vi "SMU calibration_Auto.vi"() -> ()   [LabVIEW 2020]
uses:
  <instrlib>/Keithley 2600 Series/Public/Channel.ctl
  <vilib>/Instr/_visa.llb/VISA Configure Serial Port (Instr).vi
  <vilib>/Utility/file.llb/Read Delimited Spreadsheet (DBL).vi
  <instrlib>/Keithley 2600 Series/Keithley 2600 Series.lvlib
panel:
  out "FILE":string
  out "concatenated string":string
  out "concatenated string 4":string
  out "concatenated string 3":string
  out "concatenated string 2":string
  in  "stop":bool
  in  "Tab Control":enum32{"CONTROL", "CALIBRATION"}(tab)
  in  "String":string
  in  "set En":bool
  in  "Ring":u16(ring)=1 items=["Channel 1"=1, "Channel 2"=2, "Channel 3"=3, "Channel 4"=4]
  in  "Enable 2":bool
  out "Write \nmode":bool
  in  "Mode":bool
  in  "set mode":bool
  in  "set range":bool
  in  "Range 2":u16(ring) items=["1A", "100mA", "10mA", "1mA", "100uA", "10uA", "1uA"]
  in  "set Output":bool
  in  "Output Value":dbl format="%.3f"
  out "Unit":string
  in  "set Input":bool
  in  "Level":dbl
  out "2604B \nmode":bool
  out "Array":T1(array[cluster]) {"Output level" format="%.7f"; "Voltage" format="%.7f"; "Measurement" format="%.7f"}
  in  "VISA resource \nESP(COM4)":refnum<visa-resource-name>="COM4"
  out "calibration \nmode":bool
  in  "VISA resource \n2000(COM7)":refnum<visa-resource-name>="COM7"
  in  "VISA resource \n2604B(COM8)":refnum<visa-resource-name>="COM7"
  in  "Output File calibration":bool
  in  "Output Calibration parameter path":path
  out "Output calibration parameter":string
  out "OUTPUT_F\nmode":bool
  in  "Output FIle \nCalibation Channel":u16(ring)=1 items=["Channel 1"=1, "Channel 2"=2, "Channel 3"=3, "Channel 4"=4]
  in  "Input File calibration":bool
  in  "Input Calibration parameter path  - Voltage":path
  out "Input calibration parameter":string
  out "INPUT_F\nmode":bool
  in  "Input FIle \nCalibation Channel":u16(ring)=1 items=["Channel 1"=1, "Channel 2"=2, "Channel 3"=3, "Channel 4"=4]
  in  "Input Calibration parameter path  - Current":path
  out "CH1 Calibration TX":string
  out "CH2 Calibration TX":string
  out "CH3 Calibration TX":string
  out "CH4 Calibration TX":string
  out "CH1\nCali mode":bool
  out "CH4\nCali mode":bool
  in  "calibration 4":bool
  out "CH3\nCali mode":bool
  in  "calibration 3":bool
  out "CH2\nCali mode":bool
  in  "calibration 2":bool
  in  "calibration 1":bool
  in  "Channel (Channel A)":T2
  out "STOP LED":bool
  out "tmp data":string
  out "Array 3":bool[](array[boolean])
  out "Array 2":i32[](array[numeric])
  out "test":bool
  out "extra buffer":string
  out "Range":string
  out "VI mode":string
  out "Enable":string
  out "Current":dbl
  out "Voltage":dbl
  out "Output level":dbl
  out "SMU Channel":string
  # "made by Ji Won Kim  2021.03.16"
  # "SOURCE MEASUREMENT SYSTEM"
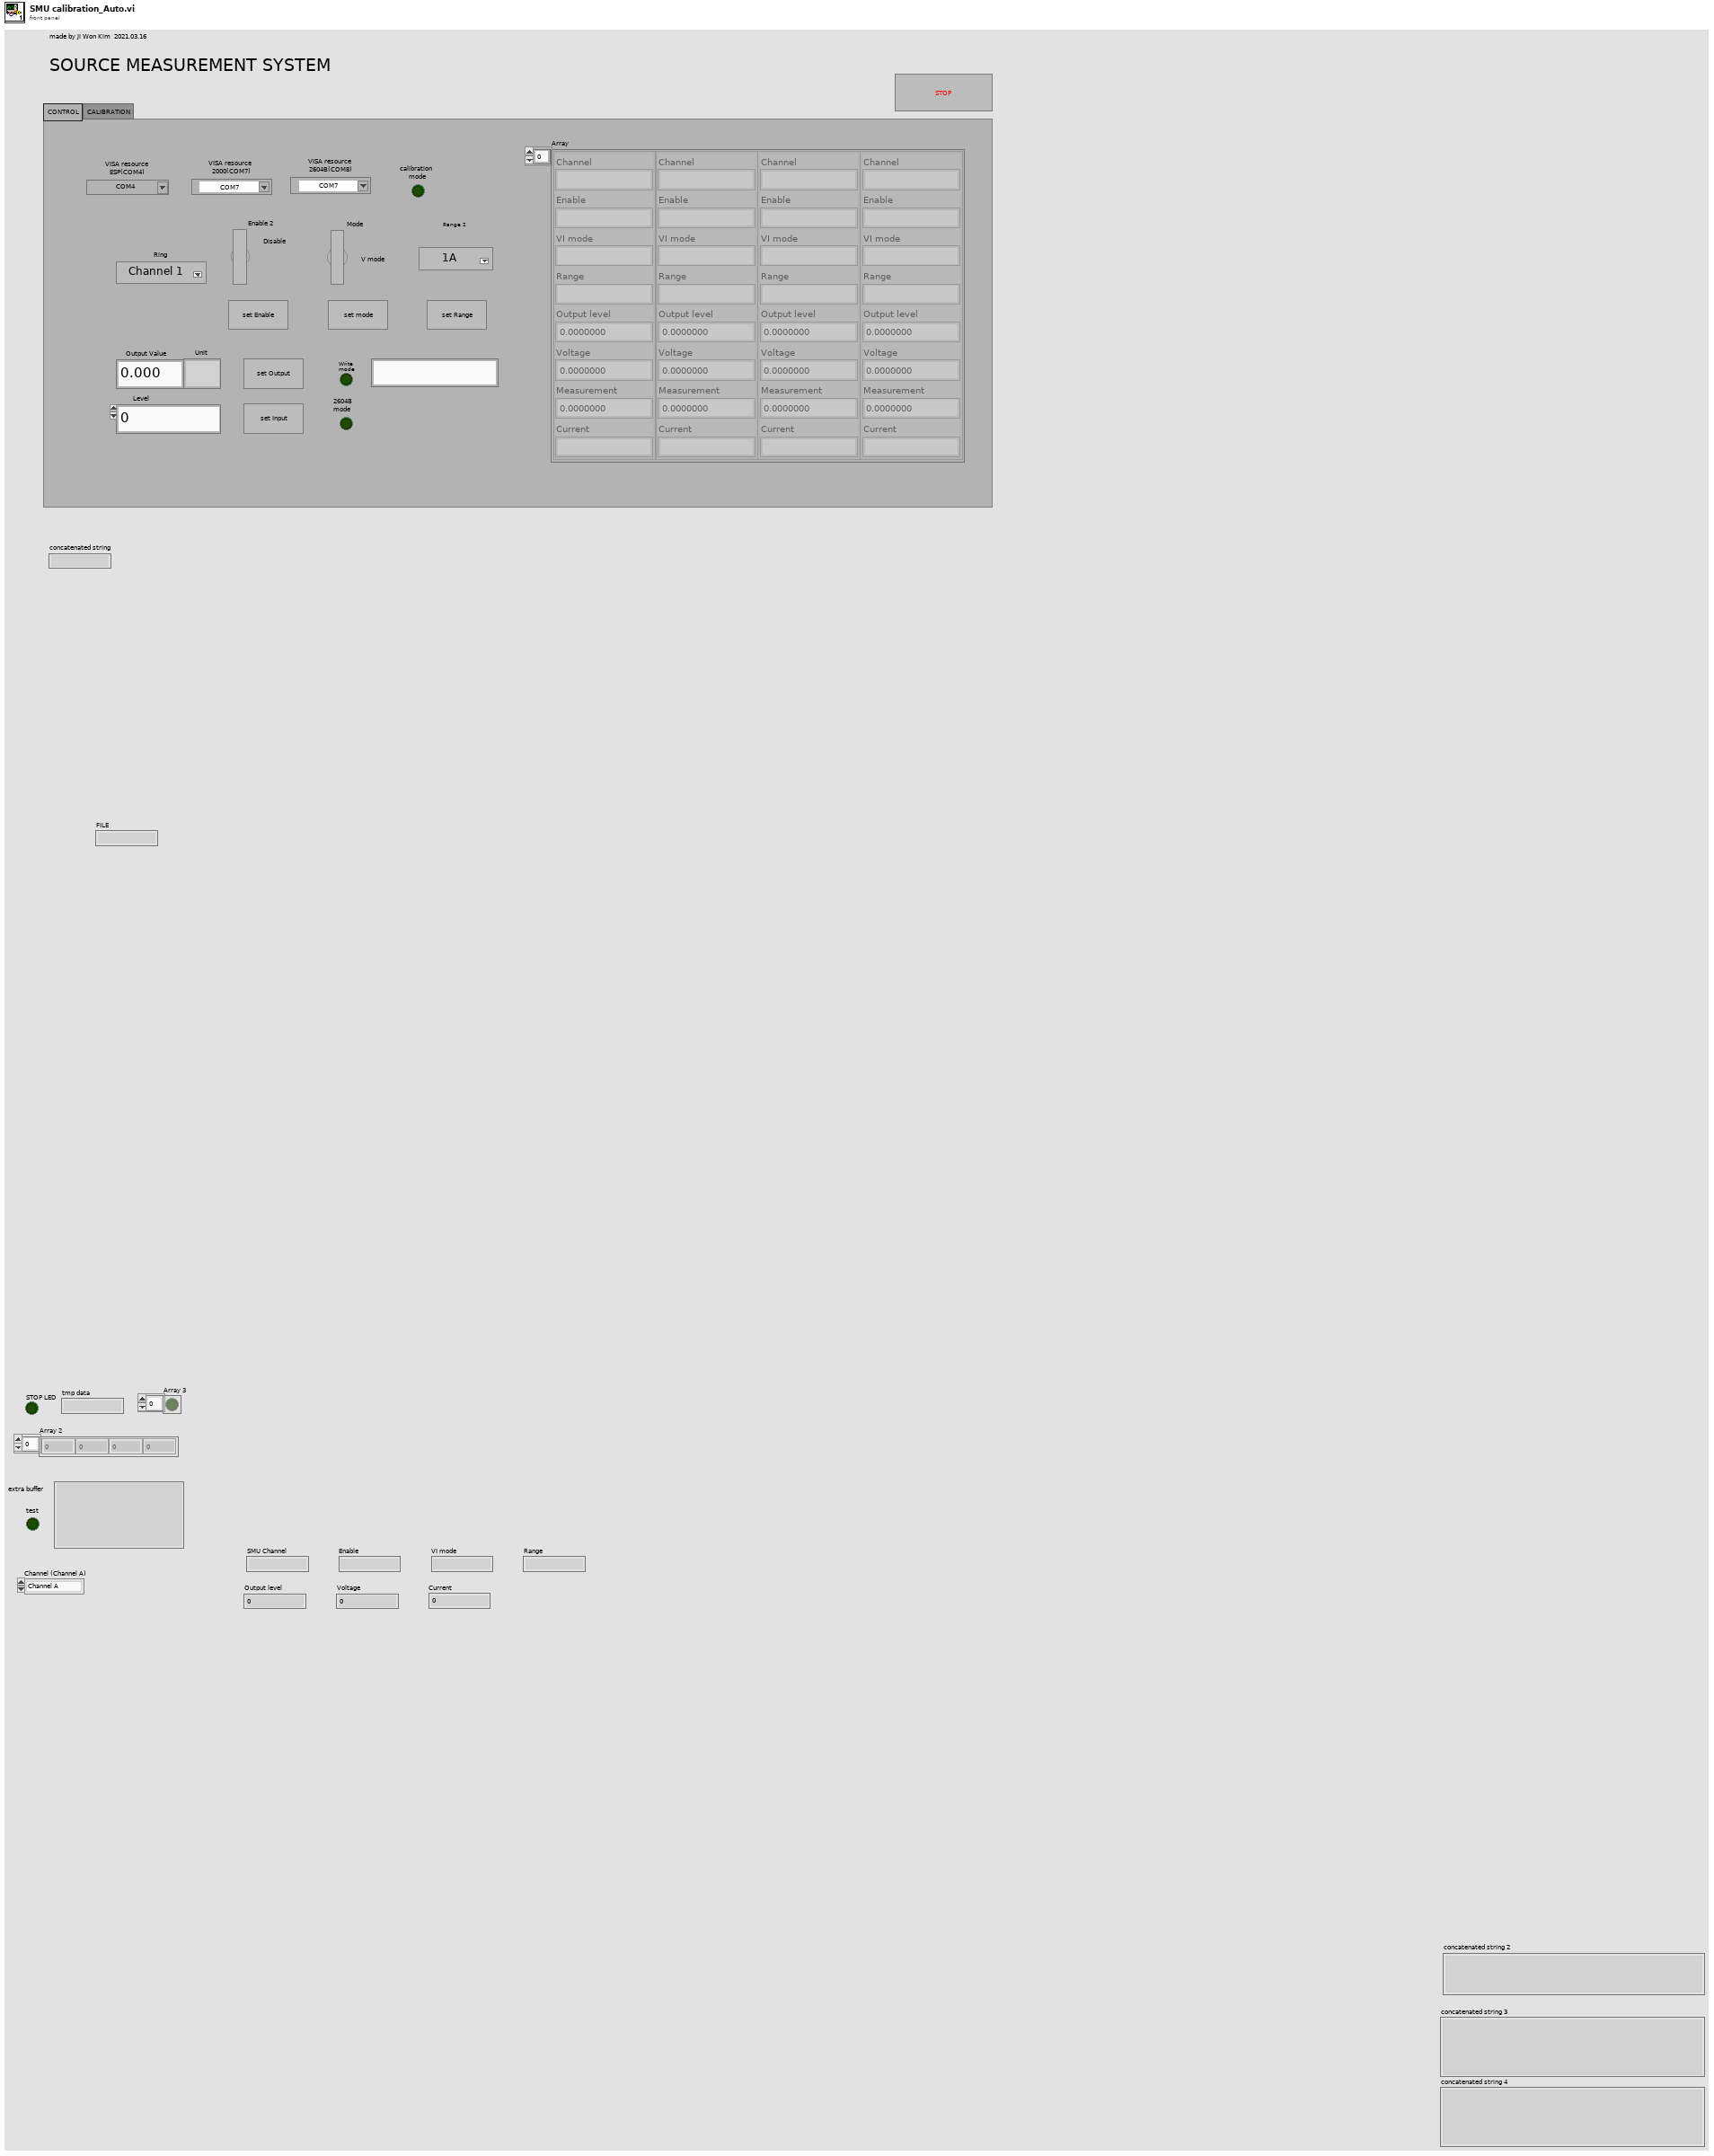
[diagram p1: front panel]
types:
  T1 = cluster{"Channel":string, "Enable":string, "VI mode":string, "Range":string, "Output level":dbl, "Voltage":dbl, "Measurement":dbl, "Current":string}[]
  T2 = typedef "Keithley 2600 Series.lvlib/Channel.ctl" = enum32{"Channel A", "Channel B"}
  T3 = cluster{"Baud Rate":u32, "Parity":u16, "Data Bits":u16, "Stop Bits":u16, "Flow Control":u16}
  T4 = cluster{"trimmed string":string, "Enable":string, "VI mode":string, "output string":string, dbl, dbl, dbl, string}
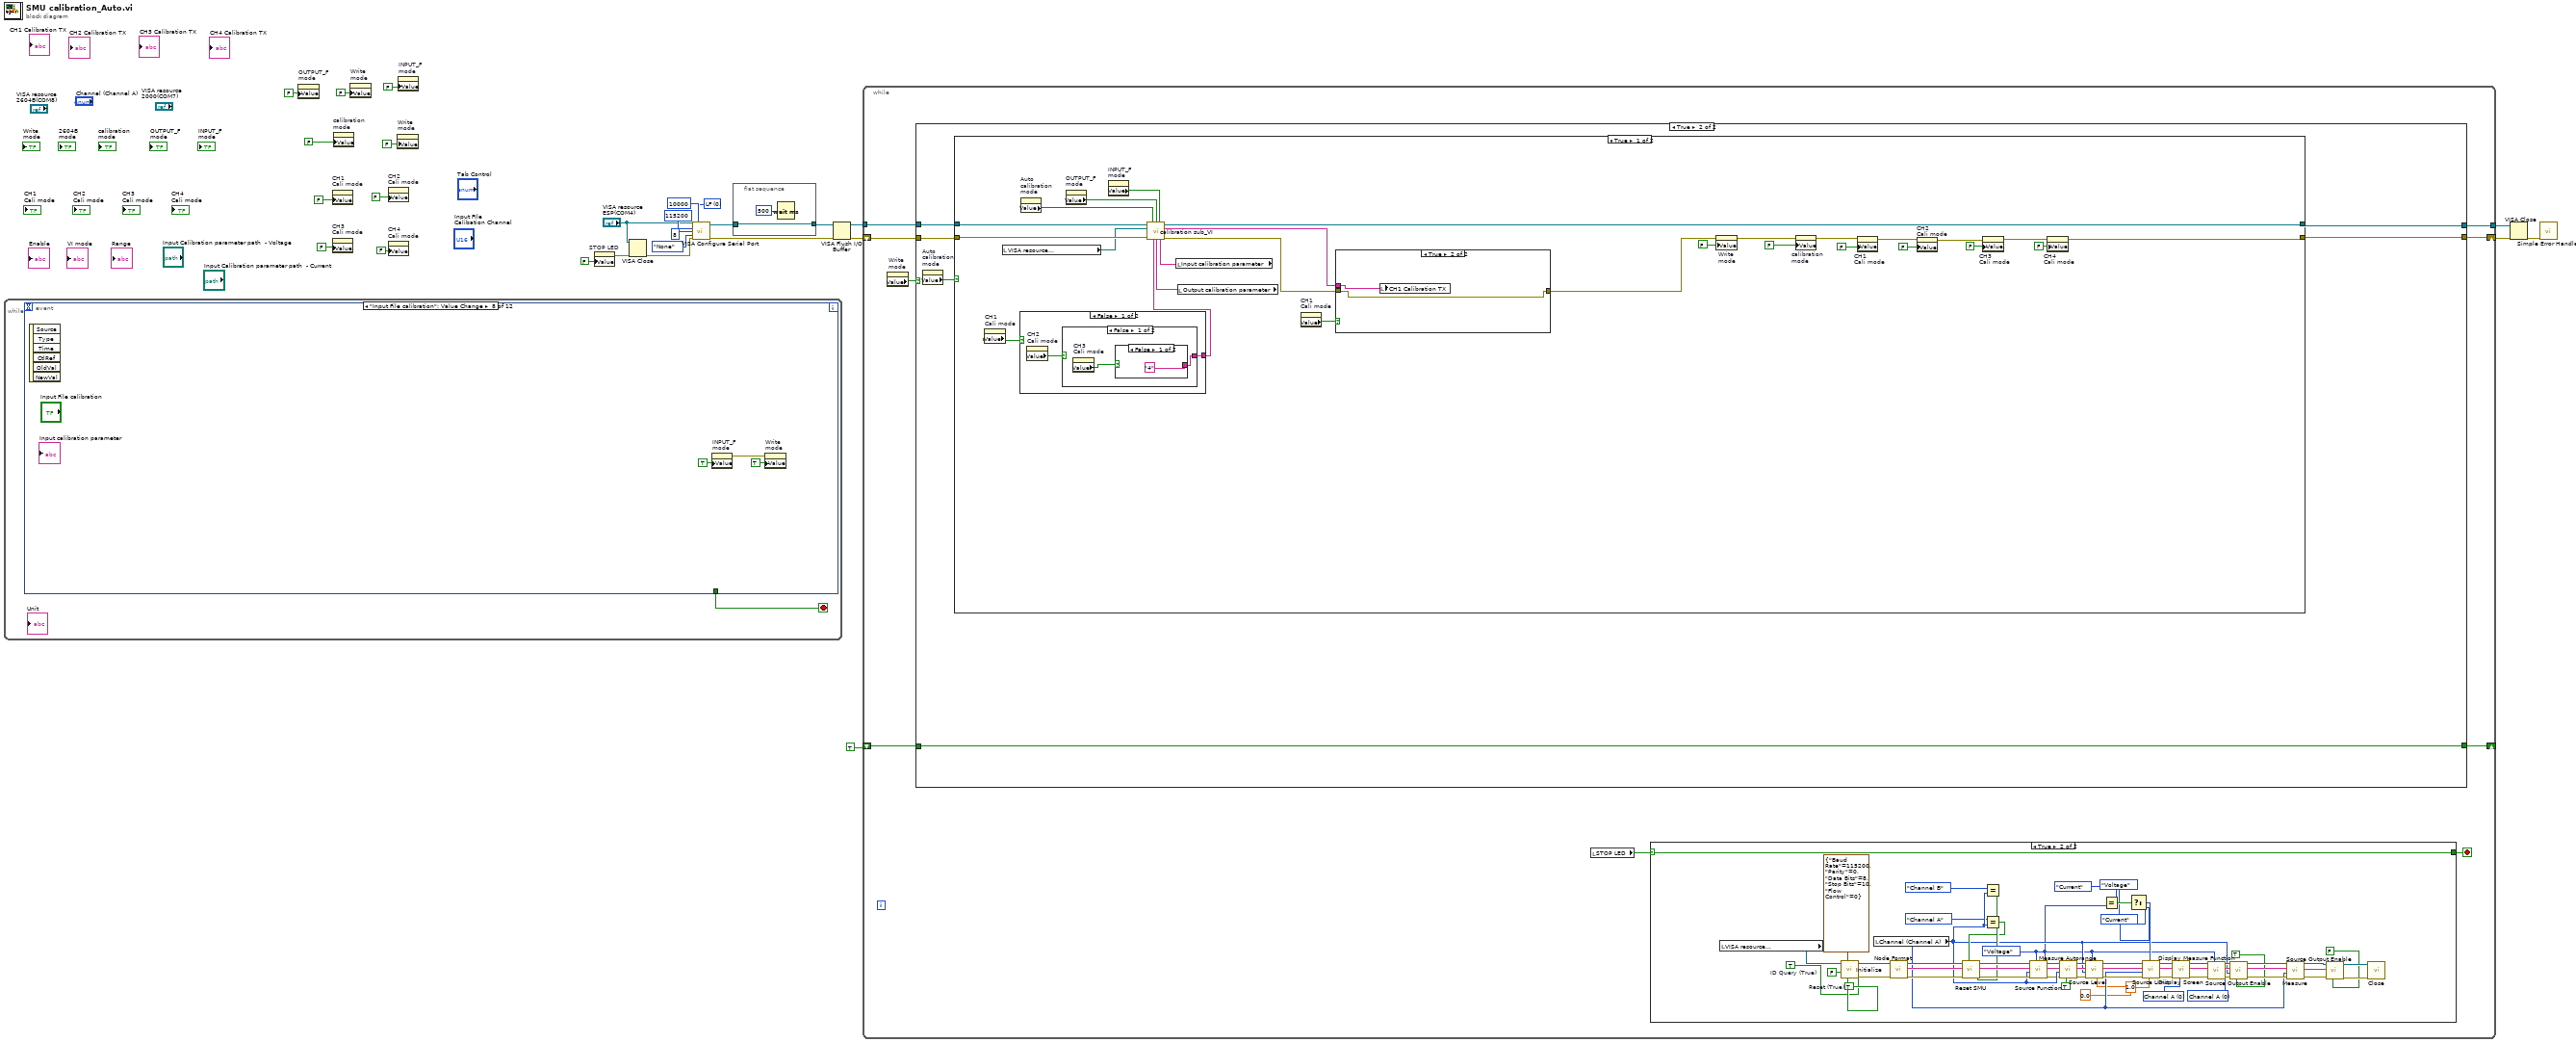
[diagram p0: block diagram]
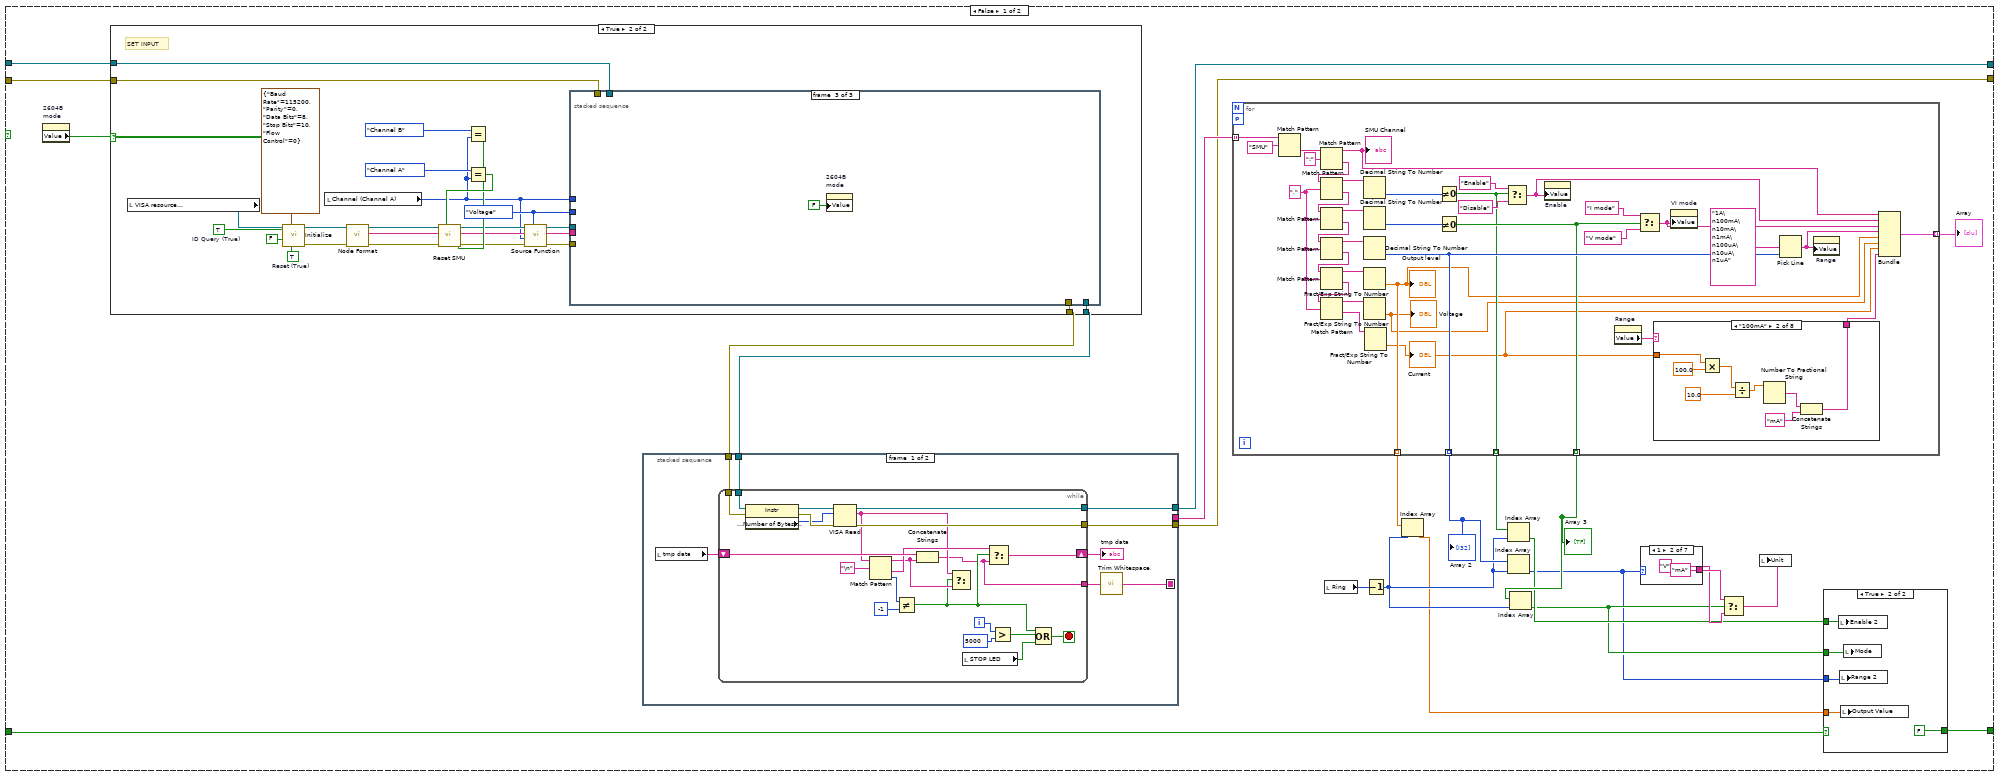
[diagram p2: hidden frame]
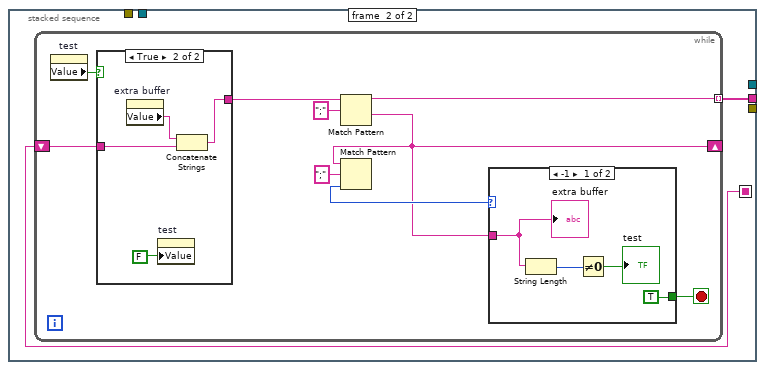
[diagram p3: hidden frame]
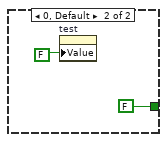
[diagram p5: hidden frame]
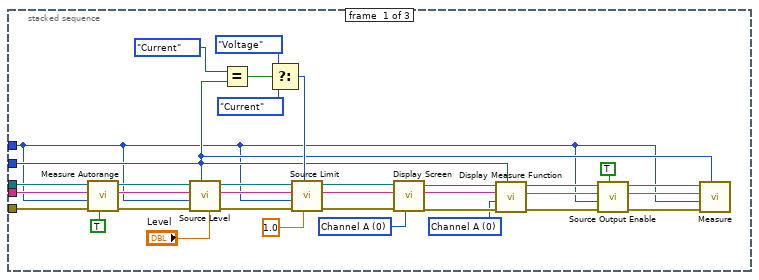
[diagram p7: hidden frame]
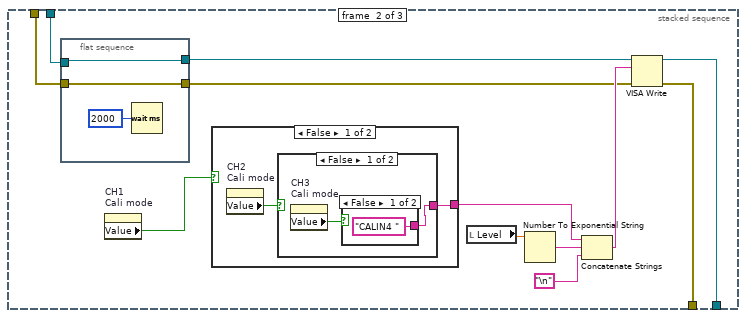
[diagram p8: hidden frame]
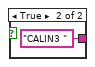
[diagram p9: hidden frame]
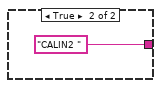
[diagram p10: hidden frame]
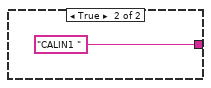
[diagram p11: hidden frame]
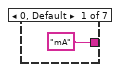
[diagram p13: hidden frame]
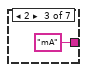
[diagram p14: hidden frame]
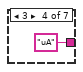
[diagram p15: hidden frame]
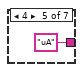
[diagram p16: hidden frame]
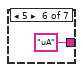
[diagram p17: hidden frame]
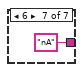
[diagram p18: hidden frame]
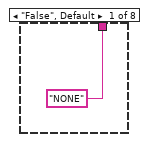
[diagram p19: hidden frame]
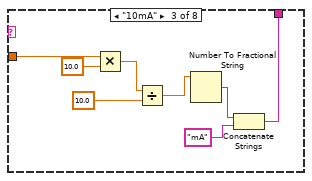
[diagram p20: hidden frame]
diagram:
  w25 = u16 0 items=["LF"]
  n1 = while {
    stop <- w28 stop-if-true
    n2 = event shown="[7] \"Input File calibration\": Value Change" {
      selector: _ -> [_ _ _ _ _ _ _ _ _ _ _ _]
      dyn-events: _ -> [_ _ _ _ _ _ _ _ _ _ _ _]
      timeout: _ -> [_ _ _ _ _ _ _ _ _ _ _ _]
      tunnel: [w29 _ _ _ _ _ _ _ _ _ _ _] -> w28
      event "stop": Value Change {
        n3 = event-data() -> ("NewVal"=w29:bool)  [unwired: 1 in, 5 out]
        "STOP LED" <- w29
      }
      event "set En": Value Change {
        n4 = event-data() -> ()  [unwired: 1 in, 6 out]
        n5 = Boolean To (0,1)(Boolean="Enable 2") -> (0, 1=w41:i16)
        n6 = Number To Decimal String(number="Ring", width (-)=i16 1) -> (decimal integer string=w39:string)
        n7 = Number To Decimal String(number=w41, width (-)=i16 1) -> (decimal integer string=w42:string)
        n8 = Concatenate Strings("ENA", w39, " " ("string"), w42, "\n") -> (w30:string)
        n9 = property on="String" class="Str"("Value"=w30) -> (error out=w32:errorcluster)  [unwired: 2 in, 1 out]
        n10 = property on="Write \nmode" class="Bool (strict)"(error in=w32, "Value"=TRUE ("Write mode")) -> ()  [unwired: 1 in, 2 out]
      }
      event "set mode": Value Change {
        n11 = event-data() -> ()  [unwired: 1 in, 6 out]
        n12 = local read "Ring"() -> (w55:u16)
        n13 = Boolean To (0,1)(Boolean="Mode") -> (0, 1=w53:i16)
        n14 = Number To Decimal String(number=w55, width (-)=i16 1) -> (decimal integer string=w51:string)
        n15 = Number To Decimal String(number=w53, width (-)=i16 1) -> (decimal integer string=w54:string)
        n16 = Concatenate Strings("VIM", w51, " " ("string"), w54, "\n") -> (w49:string)
        n17 = property on="String" class="Str"("Value"=w49) -> (error out=w50:errorcluster)  [unwired: 2 in, 1 out]
        n18 = property on="Write \nmode" class="Bool (strict)"(error in=w50, "Value"=TRUE ("Write mode")) -> ()  [unwired: 1 in, 2 out]
      }
      event "set range": Value Change {
        n19 = event-data() -> ()  [unwired: 1 in, 6 out]
        n20 = local read "Ring"() -> (w66:u16)
        n21 = Number To Decimal String(number=w66, width (-)=i16 1) -> (decimal integer string=w64:string)
        n22 = Number To Decimal String(number="Range 2", width (-)=i16 1) -> (decimal integer string=w65:string)
        n23 = Concatenate Strings("RAN", w64, " " ("string"), w65, "\n") -> (w62:string)
        n24 = property on="String" class="Str"("Value"=w62) -> (error out=w63:errorcluster)  [unwired: 2 in, 1 out]
        n25 = property on="Write \nmode" class="Bool (strict)"(error in=w63, "Value"=TRUE ("Write mode")) -> ()  [unwired: 1 in, 2 out]
      }
      event "set Output": Value Change {
        n26 = event-data() -> ()  [unwired: 1 in, 6 out]
        n27 = local read "Ring"() -> (w76:u16)
        n28 = local read "Array 2"() -> (w75:i32[])
        n29 = Decrement(x=w76) -> (x-1=w69:u16)
        n30 = Index Array(array=w75, index=w69) -> (element=w74:i32)
        n31 = case shown="0, Default" w74 {
          tunnel: [1000.0 100.0 10.0 1000.0 100.0 10.0 1.0] -> w77
          frame 0, Default {
          }
          frame 1 {
          }
          frame 2 {
          }
          frame 3 {
          }
          frame 4 {
          }
          frame 5 {
          }
          frame 6 {
          }
        }
        n32 = local read "Array 3"() -> (w71:bool[])
        n33 = Index Array(array=w71, index=w69) -> (element=w70:bool)
        n34 = Divide(x="Output Value", y=w77) -> (x/y=w78:dbl)
        n35 = Multiply(x=w78, y=10.0) -> (x*y=w73:dbl)
        n36 = Select(t=w73, s=w70, f="Output Value") -> (s? t:f=w68:dbl)
        n37 = local read "Ring"() -> (w89:u16)
        n38 = Number To Fractional String(number=w68, precision (6)=i16 4) -> (F-format string=w90:string)  [unwired: 2 in]
        n39 = Number To Decimal String(number=w89, width (-)=i16 1) -> (decimal integer string=w88:string)
        n40 = Concatenate Strings("CAL", w88, " " ("string"), w90, "\n") -> (w86:string)
        n41 = property on="String" class="Str"("Value"=w86) -> (error out=w87:errorcluster)  [unwired: 2 in, 1 out]
        n42 = property on="Write \nmode" class="Bool (strict)"(error in=w87, "Value"=TRUE ("Write mode")) -> ()  [unwired: 1 in, 2 out]
      }
      event "set Input": Value Change {
        n43 = event-data() -> ()  [unwired: 1 in, 6 out]
        n44 = property on="2604B \nmode" class="Bool (strict)"("Value"=TRUE ("2604B mode")) -> ()  [unwired: 2 in, 2 out]
      }
      event "Output File calibration": Value Change {
        n45 = event-data() -> ()  [unwired: 1 in, 6 out]
        n46 = call-poly <vilib>:"Read Delimited Spreadsheet.vi"("file path (dialog if empty)"="Output Calibration parameter path", "delimiter (\\t)"="," ("delimiter (\\t)")) -> ("all rows"=w111:dbl[][])  [unwired: 8 in, 5 out]
        n47 = Index Array(array=w111, index (col)=1 ("disabled index (col)")) -> (element=w115:dbl[])  [unwired: 1 in]
        n48 = Array To Spreadsheet String(delimiter (Tab)=",", array=w115, 3:"%5.3f" ("format string")) -> (spreadsheet string=w109:string)
        n49 = Number To Decimal String(number="Output FIle \nCalibation Channel", width (-)=i16 1) -> (decimal integer string=w100:string)
        n50 = call <vilib>:"Trim Whitespace.vi"("string"=w109) -> ("trimmed string"=w108:string)  [unwired: 1 in]
        n51 = Concatenate Strings("DAQ" ("string"), w100, " " ("string"), "-10,-9,-8,-7,-6,-5,-4,-3,-2,-1,0,1,2,3,4,5,6,7,8,9,10" ("string"), ";" ("string"), w108, "\n") -> (w107:string)
        n52 = Concatenate Strings(w107, "\n") -> (w118:string)
        n53 = property on="Output calibration parameter" class="Str"("Value"=w118) -> (error out=w121:errorcluster)  [unwired: 2 in, 1 out]
        n54 = property on="OUTPUT_F\nmode" class="Bool (strict)"(error in=w121, "Value"=TRUE ("calibration mode 2")) -> (error out=w119:errorcluster)  [unwired: 1 in, 1 out]
        n55 = property on="Write \nmode" class="Bool (strict)"(error in=w119, "Value"=TRUE ("Write mode")) -> ()  [unwired: 1 in, 2 out]
      }
      event "Input File calibration": Value Change {
        n56 = event-data() -> ()  [unwired: 1 in, 6 out]
        n57 = property on="INPUT_F\nmode" class="Bool (strict)"("Value"=TRUE ("calibration mode 2")) -> (error out=w123:errorcluster)  [unwired: 2 in, 1 out]
        n58 = property on="Write \nmode" class="Bool (strict)"(error in=w123, "Value"=TRUE ("Write mode")) -> ()  [unwired: 1 in, 2 out]
      }
      event "calibration 1": Value Change {
        n59 = event-data() -> ()  [unwired: 1 in, 6 out]
        n60 = property on="calibration \nmode" class="Bool (strict)"("Value"=TRUE ("Write mode")) -> (error out=w128:errorcluster)  [unwired: 2 in, 1 out]
        n61 = property on="Write \nmode" class="Bool (strict)"(error in=w128, "Value"=TRUE ("Write mode")) -> (error out=w127:errorcluster)  [unwired: 1 in, 1 out]
        n62 = property on="CH1\nCali mode" class="Bool (strict)"(error in=w127, "Value"=TRUE ("Write mode")) -> ()  [unwired: 1 in, 2 out]
      }
      event "calibration 2": Value Change {
        n63 = event-data() -> ()  [unwired: 1 in, 6 out]
        n64 = property on="calibration \nmode" class="Bool (strict)"("Value"=TRUE ("Write mode")) -> (error out=w133:errorcluster)  [unwired: 2 in, 1 out]
        n65 = property on="Write \nmode" class="Bool (strict)"(error in=w133, "Value"=TRUE ("Write mode")) -> (error out=w132:errorcluster)  [unwired: 1 in, 1 out]
        n66 = property on="CH2\nCali mode" class="Bool (strict)"(error in=w132, "Value"=TRUE ("Write mode")) -> ()  [unwired: 1 in, 2 out]
      }
      event "calibration 3": Value Change {
        n67 = event-data() -> ()  [unwired: 1 in, 6 out]
        n68 = property on="calibration \nmode" class="Bool (strict)"("Value"=TRUE ("Write mode")) -> (error out=w138:errorcluster)  [unwired: 2 in, 1 out]
        n69 = property on="Write \nmode" class="Bool (strict)"(error in=w138, "Value"=TRUE ("Write mode")) -> (error out=w137:errorcluster)  [unwired: 1 in, 1 out]
        n70 = property on="CH3\nCali mode" class="Bool (strict)"(error in=w137, "Value"=TRUE ("Write mode")) -> ()  [unwired: 1 in, 2 out]
      }
      event "calibration 4": Value Change {
        n71 = event-data() -> ()  [unwired: 1 in, 6 out]
        n72 = property on="calibration \nmode" class="Bool (strict)"("Value"=TRUE ("Write mode")) -> (error out=w143:errorcluster)  [unwired: 2 in, 1 out]
        n73 = property on="Write \nmode" class="Bool (strict)"(error in=w143, "Value"=TRUE ("Write mode")) -> (error out=w142:errorcluster)  [unwired: 1 in, 1 out]
        n74 = property on="CH4\nCali mode" class="Bool (strict)"(error in=w142, "Value"=TRUE ("Write mode")) -> ()  [unwired: 1 in, 2 out]
      }
    }
  }
  n75 = property on="OUTPUT_F\nmode" class="Bool (strict)"("Value"=FALSE ("calibration mode 2")) -> ()  [unwired: 2 in, 2 out]
  n76 = property on="CH1\nCali mode" class="Bool (strict)"("Value"=FALSE ("Write mode")) -> ()  [unwired: 2 in, 2 out]
  n77 = property on="CH3\nCali mode" class="Bool (strict)"("Value"=FALSE ("calibration \nmode 3")) -> ()  [unwired: 2 in, 2 out]
  n78 = property on="calibration \nmode" class="Bool (strict)"("Value"=FALSE ("calibration mode")) -> ()  [unwired: 2 in, 2 out]
  n79 = property on="Write \nmode" class="Bool (strict)"("Value"=FALSE ("Write mode")) -> ()  [unwired: 2 in, 2 out]
  n80 = property on="CH2\nCali mode" class="Bool (strict)"("Value"=FALSE ("calibration \nmode 2")) -> ()  [unwired: 2 in, 2 out]
  n81 = property on="CH4\nCali mode" class="Bool (strict)"("Value"=FALSE ("calibration \nmode 4")) -> ()  [unwired: 2 in, 2 out]
  n82 = property on="Write \nmode" class="Bool (strict)"("Value"=FALSE ("Write mode")) -> ()  [unwired: 2 in, 2 out]
  n83 = property on="INPUT_F\nmode" class="Bool (strict)"("Value"=FALSE ("Write mode")) -> ()  [unwired: 2 in, 2 out]
  n84 = property on="STOP LED" class="Bool (strict)"("Value"=FALSE ("NewVal")) -> (error out=w11:errorcluster)  [unwired: 2 in, 1 out]
  n85 = VISA Close(VISA resource name="VISA resource \nESP(COM4)", error in (no error)=w11) -> (error out=w13:errorcluster)
  n86 = call-poly "VISA Configure Serial Port"("VISA resource name"="VISA resource \nESP(COM4)", "timeout (10sec)"=u32 10000, "termination char\n(0xA = '\\n' = LF)"=w25, "baud rate (9600)"=u32 115200, "data bits (8)"=u16 8, "parity (0:none)"=enum16{"None", "Odd", "Even", "Mark", "Space"}."None", "error in (no error)"=w13) -> ("VISA resource name out"=w19:refnum<visa-resource-name>, "error out"=w17:errorcluster)  [unwired: 7 in]
  n87 = flat-sequence {
    tunnel: [w146] -> w18
    tunnel: w19 -> [w146]
    frame #0 {
      n88 = Wait (ms)(milliseconds to wait=u32 500 ("대기 시간(ms)")) -> ()  [unwired: 1 out]
    }
  }
  n89 = VISA Flush I/O Buffer(VISA resource name=w18, error in (no error)=w17) -> (VISA resource name out=w15:refnum<visa-resource-name>, error out=w16:errorcluster)  [unwired: 1 in]
  n90 = while {
    tunnel: [w156] -> w27
    shift-right: [w152] -> w21
    shift-left: w16 -> [w151]
    tunnel: w15 -> [w155]
    shift-right: [w153] -> _
    shift-left: TRUE -> [w154]
    stop <- w149 stop-if-true
    n91 = property on="Write \nmode" class="Bool (strict)"() -> ("Value"=w148:bool)  [unwired: 2 in, 2 out]
    n92 = case shown="True" w148 {
      tunnel: [w157 w427] -> w152
      tunnel: [w158 w428] -> w156
      tunnel: w155 -> [w164 w429]
      tunnel: w154 -> [w167 w426]
      tunnel: [w166 w426] -> w153
      tunnel: w151 -> [w163 w424]
      frame False {
        n93 = property on="2604B \nmode" class="Bool (strict)"() -> ("Value"=w162:bool)  [unwired: 2 in, 2 out]
        n94 = case shown="True" w162 {
          tunnel: w164 -> [w234 w259]
          tunnel: w163 -> [w233 w258]
          tunnel: [w234 w235] -> w160
          tunnel: [w233 w236] -> w161
          frame False {
          }
          frame True {
            w240 = enum32{"Current", "Voltage"}."Voltage" ("Source Function (Current)")
            w256 = TRUE  # Reset (True)
            w257 = TRUE  # ID Query (True)
            # "SET INPUT"
            n95 = local read "VISA resource \n2604B(COM8)"() -> (w238:refnum<visa-resource-name>)
            n96 = call <instrlib>:"Initialize.vi"("Reset (True)"=w256, "Serial Configuration"=T3 {"Baud Rate"=115200, "Parity"=0, "Data Bits"=8, "Stop Bits"=10, "Flow Control"=0}, "Error Query (False)"=FALSE, "ID Query (True)"=w257, "VISA resource name"=w238) -> ("error out"=w245:errorcluster, "VISA resource name out"=w254:refnum<visa-resource-name>)  [unwired: 1 in, 4 out]
            n97 = local read "Channel (Channel A)"() -> (w237:T2)
            n98 = call <instrlib>:"Node Format.vi"("error in"=w245) -> ("error out"=w244:errorcluster, "Formatted Node"=w246:string)  [unwired: 1 in, 8 out]
            n99 = Equal?(x=enum32{"Channel A", "Channel B"}."Channel B", y=w237) -> (x = y?=w250:bool)
            n100 = Equal?(x=enum32{"Channel A", "Channel B"}."Channel A", y=w237) -> (x = y?=w251:bool)
            n101 = call <instrlib>:"Reset SMU.vi"("SMU B (No)"=w250, "SMU A (No)"=w251, "error in (no error)"=w244, "Node In"=w246, "VISA resource name"=w254) -> ("error out"=w249:errorcluster, "Node Out"=w247:string, "VISA resource name out"=w248:refnum<visa-resource-name>)  [unwired: 4 out]
            n102 = call <instrlib>:"Source Function.vi"("Function (Current)"=w240, "error in (no error)"=w249, "Channel (Channel A)"=w237, "Node In"=w247, "VISA resource name"=w248) -> ("error out"=w241:errorcluster, "Node Out"=w243:string, "VISA resource name out"=w242:refnum<visa-resource-name>)  [unwired: 4 out]
            n103 = stacked-sequence {
              tunnel: w243 -> [w264 _ _]
              tunnel: w242 -> [w267 _ _]
              tunnel: w241 -> [w263 _ _]
              tunnel: w237 -> [w261 _ _]
              tunnel: w240 -> [w270 _ _]
              tunnel: w259 -> [_ w305 _]
              tunnel: w258 -> [_ w304 _]
              tunnel: [_ w297 _] -> w235
              tunnel: [_ w296 _] -> w236
              frame #0 {
                w271 = u16 0 items=["Channel A", "Channel B"] ("Channel (Channel A)")
                w281 = u16 0 items=["Channel A", "Channel B", "Channels A & B", "User"] ("Screen (Channels A & B)")
                n104 = call <instrlib>:"Measure Autorange.vi"("Autorange (On)"=TRUE, "error in (no error)"=w263, "Channel (Channel A)"=w261, "Node In"=w264, "VISA resource name"=w267) -> ("error out"=w262:errorcluster, "Node Out"=w265:string, "VISA resource name out"=w266:refnum<visa-resource-name>)  [unwired: 3 in, 1 out]
                n105 = call <instrlib>:"Source Level.vi"("Level (0.000)"="Level", "Function (Current)"=w270, "error in (no error)"=w262, "Channel (Channel A)"=w261, "Node In"=w265, "VISA resource name"=w266) -> ("error out"=w293:errorcluster, "Node Out"=w288:string, "VISA resource name out"=w292:refnum<visa-resource-name>)  [unwired: 3 out]
                n106 = Equal?(x=enum32{"Current", "Voltage"}."Current", y=w270) -> (x = y?=w285:bool)
                n107 = Select(t=enum32{"Current", "Voltage"}."Voltage" ("x"), s=w285, f=enum32{"Current", "Voltage"}."Current") -> (s? t:f=w283:enum32{"Current", "Voltage"})
                n108 = call <instrlib>:"Source Limit.vi"("Limit (0.000)"=1.0, "Function (Current)"=w283, "error in (no error)"=w293, "Channel (Channel A)"=w261, "Node In"=w288, "VISA resource name"=w292) -> ("error out"=w278:errorcluster, "Node Out"=w279:string, "VISA resource name out"=w280:refnum<visa-resource-name>)  [unwired: 3 out]
                n109 = call <instrlib>:"Display Screen.vi"("Screen (Channels A & B)"=w281, "error in (no error)"=w278, "Node In"=w279, "VISA resource name"=w280) -> ("error out"=w275:errorcluster, "Node Out"=w276:string, "VISA resource name out"=w277:refnum<visa-resource-name>)  [unwired: 4 in, 1 out]
                n110 = call <instrlib>:"Display Measure Function.vi"("Function (Current)"=w270, "error in (no error)"=w275, "Channel (Channel A)"=w271, "Node In"=w276, "VISA resource name"=w277) -> ("error out"=w272:errorcluster, "Node Out"=w273:string, "VISA resource name out"=w274:refnum<visa-resource-name>)  [unwired: 3 in, 1 out]
                n111 = call <instrlib>:"Source Output Enable.vi"("Output (Off)"=TRUE, "error in (no error)"=w272, "Channel (Channel A)"=w261, "Node In"=w273, "VISA resource name"=w274) -> ("error out"=w291:errorcluster, "Node Out"=w287:string, "VISA resource name out"=w290:refnum<visa-resource-name>)  [unwired: 4 out]
                n112 = call <instrlib>:"Measure.vi"("Function (Current)"=w270, "error in (no error)"=w291, "Channel (Channel A)"=w261, "Node In"=w287, "VISA resource name"=w290) -> ()  [unwired: 2 in, 5 out]
              }
              frame #1 {
                n113 = flat-sequence {
                  tunnel: w305 -> [w316]
                  tunnel: [w316] -> w299
                  tunnel: w304 -> [w315]
                  tunnel: [w315] -> w298
                  frame #0 {
                    n114 = Wait (ms)(milliseconds to wait=u32 2000) -> ()  [unwired: 1 out]
                  }
                }
                n115 = property on="CH1\nCali mode" class="Bool (strict)"() -> ("Value"=w295:bool)  [unwired: 2 in, 2 out]
                n116 = case shown="False" w295 {
                  tunnel: [w306 "CALIN1 " ("string")] -> w294
                  frame False {
                    n117 = property on="CH2\nCali mode" class="Bool (strict)"() -> ("Value"=w307:bool)  [unwired: 2 in, 2 out]
                    n118 = case shown="False" w307 {
                      tunnel: [w308 "CALIN2 " ("string")] -> w306
                      frame False {
                        n119 = property on="CH3\nCali mode" class="Bool (strict)"() -> ("Value"=w309:bool)  [unwired: 2 in, 2 out]
                        n120 = case shown="False" w309 {
                          tunnel: ["CALIN4 " ("string") "CALIN3 " ("string")] -> w308
                          frame False {
                          }
                          frame True {
                          }
                        }
                      }
                      frame True {
                      }
                    }
                  }
                  frame True {
                  }
                }
                n121 = local read "Level"() -> (w303:dbl)
                n122 = Number To Exponential String(number=w303) -> (E-format string=w300:string)  [unwired: 3 in]
                n123 = Concatenate Strings(w294, w300, "\n") -> (w302:string)
                n124 = VISA Write(VISA resource name=w299, write buffer=w302, error in (no error)=w298) -> (VISA resource name out=w297:refnum<visa-resource-name>, error out=w296:errorcluster)  [unwired: 1 out]
              }
              frame #2 {
                n125 = property on="2604B \nmode" class="Bool (strict)"("Value"=FALSE ("2604B mode")) -> ()  [unwired: 2 in, 2 out]
              }
            }
          }
        }
        n126 = stacked-sequence {
          seq-local: [w183 _] -> [_ w212]
          tunnel: w161 -> [w184 _]
          tunnel: w160 -> [w185 _]
          tunnel: [_ w211] -> w159
          tunnel: [w182 _] -> w158
          tunnel: [w181 _] -> w157
          frame #0 {
            n127 = local read "tmp data"() -> (w186:string)
            n128 = while {
              tunnel: [w210] -> w181
              tunnel: [w209] -> w182
              shift-right: [w200] -> w187
              shift-left: w186 -> [w204]
              tunnel: [w191] -> w188
              tunnel: w185 -> [w190]
              tunnel: w184 -> [w189]
              i -> [w196]
              stop <- w192 stop-if-true
              n129 = property class="Instr"(reference=w190, error in=w189) -> (reference out=w208:refnum<visa-resource-name>, error out=w207:errorcluster, "Serial Settings:Number of Bytes at Serial Port"=w206:u32)
              n130 = VISA Read(VISA resource name=w208, byte count=w206, error in (no error)=w207) -> (VISA resource name out=w209:refnum<visa-resource-name>, read buffer=w202:string, error out=w210:errorcluster)  [unwired: 1 out]
              n131 = Match Pattern(string=w202, regular expression="\n") -> (before substring=w201:string, after substring=w203:string, offset past match=w198:i32)  [unwired: 1 in, 1 out]
              n132 = Not Equal?(x=w198, y=-1) -> (x != y?=w195:bool)
              n133 = Concatenate Strings(w204, w201) -> (w191:string)
              n134 = Select(t=w202, s=w195, f=w201) -> ()  [unwired: 1 out]
              n135 = local read "STOP LED"() -> (w193:bool)
              n136 = Select(t=w203, s=w195, f=w191) -> (s? t:f=w200:string)
              n137 = Greater?(x=w196, y=5000) -> (0:w194:bool)
              n138 = Compound Arithmetic op=OR(w195, w194, w193) -> (w192:bool)
            }
            "tmp data" <- w187
            n139 = call <vilib>:"Trim Whitespace.vi"("string"=w188) -> ("trimmed string"=w183:string)  [unwired: 1 in]
          }
          frame #1 {
            n140 = while {
              shift-right: [w213] -> _
              shift-left: w212 -> [w216]
              tunnel: [w220] -> w211 mode=indexing
              stop <- w214 stop-if-true
              n141 = property on="test" class="Bool (strict)"() -> ("Value"=w217:bool)  [unwired: 2 in, 2 out]
              n142 = case shown="True" w217 {
                tunnel: w216 -> [w222 w225]
                tunnel: [w222 w224] -> w215
                frame False {
                }
                frame True {
                  n143 = property on="extra buffer" class="Str"() -> ("Value"=w226:string)  [unwired: 2 in, 2 out]
                  n144 = property on="test" class="Bool (strict)"("Value"=FALSE) -> ()  [unwired: 2 in, 2 out]
                  n145 = Concatenate Strings(w226, w225) -> (w224:string)
                }
              }
              n146 = Match Pattern(string=w215, regular expression=";" ("search string")) -> (before substring=w220:string, after substring=w213:string)  [unwired: 1 in, 2 out]
              n147 = Match Pattern(string=w213, regular expression=";" ("search string")) -> (offset past match=w218:i32)  [unwired: 1 in, 3 out]
              n148 = case shown="-1" w218 {
                tunnel: w213 -> [w229 _]
                tunnel: [TRUE FALSE] -> w214
                frame -1 {
                  n149 = String Length(string=w229) -> (length=w228:i32)
                  n150 = Not Equal To 0?(x=w228) -> (x != 0?=→"test":bool)
                  "extra buffer" <- w229
                }
                frame 0, Default {
                  n151 = property on="test" class="Bool (strict)"("Value"=FALSE) -> ()  [unwired: 2 in, 2 out]
                }
              }
            }
          }
        }
        n152 = for {
          tunnel: [w366] -> w165 mode=indexing
          workers-P: _ -> [_]
          tunnel: [w341] -> w179 mode=indexing
          tunnel: [w340] -> w178 mode=indexing
          tunnel: [w336] -> w174 mode=indexing
          tunnel: [w335] -> w170 mode=indexing
          tunnel: w159 -> [w334] mode=indexing
          w357 = "," ("search string")
          n153 = Match Pattern(string=w334, regular expression="SMU") -> (after substring=w363:string)  [unwired: 1 in, 3 out]
          n154 = Match Pattern(string=w363, regular expression=":" ("search string")) -> (before substring=w342:string, after substring=w362:string)  [unwired: 1 in, 2 out]
          "SMU Channel" <- w342
          n155 = Match Pattern(string=w362, regular expression=w357) -> (before substring=w356:string, after substring=w361:string)  [unwired: 1 in, 2 out]
          n156 = Match Pattern(string=w361, regular expression=w357) -> (before substring=w351:string, after substring=w359:string)  [unwired: 1 in, 2 out]
          n157 = Match Pattern(string=w359, regular expression=w357) -> (before substring=w352:string, after substring=w360:string)  [unwired: 1 in, 2 out]
          n158 = Match Pattern(string=w360, regular expression=w357) -> (before substring=w353:string, after substring=w358:string)  [unwired: 1 in, 2 out]
          n159 = Match Pattern(string=w358, regular expression=w357) -> (before substring=w354:string, after substring=w355:string)  [unwired: 1 in, 2 out]
          n160 = Decimal String To Number(string=w356) -> (number=w350:i32)  [unwired: 2 in, 1 out]
          n161 = Decimal String To Number(string=w351) -> (number=w349:i32)  [unwired: 2 in, 1 out]
          n162 = Decimal String To Number(string=w352) -> (number=w341:i32)  [unwired: 2 in, 1 out]
          n163 = Fract/Exp String To Number(string=w353) -> (number=w335:dbl)  [unwired: 3 in, 1 out]
          "Output level" <- w335
          n164 = Fract/Exp String To Number(string=w354) -> (number=w333:dbl)  [unwired: 3 in, 1 out]
          "Voltage" <- w333
          n165 = Fract/Exp String To Number(string=w355) -> (number=w332:dbl)  [unwired: 3 in, 1 out]
          "Current" <- w332
          n166 = Not Equal To 0?(x=w350) -> (x != 0?=w336:bool)
          n167 = Not Equal To 0?(x=w349) -> (x != 0?=w340:bool)
          n168 = Select(t="Enable" ("Enable"), s=w336, f="Disable" ("Enable")) -> (s? t:f=w344:string)
          n169 = property on="Enable" class="Str"("Value"=w344) -> ()  [unwired: 2 in, 2 out]
          n170 = property on="Range" class="Str"() -> ("Value"=w331:string)  [unwired: 2 in, 2 out]
          n171 = Select(t="I mode" ("VI mode"), s=w340, f="V mode" ("VI mode")) -> (s? t:f=w343:string)
          n172 = case shown="\"100mA\"" w331 {
            tunnel: ["NONE" w371 w379 w387 w395 w403 w411 w419] -> w337
            tunnel: w332 -> [_ w370 w376 w386 w394 w402 w410 w418]
            frame "False", Default {
            }
            frame "100mA" {
              n173 = Multiply(x=w370, y=100.0) -> (x*y=w374:dbl)
              n174 = Divide(x=w374, y=10.0) -> (x/y=w369:dbl)
              n175 = Number To Fractional String(number=w369) -> (F-format string=w368:string)  [unwired: 3 in]
              n176 = Concatenate Strings(w368, "mA" ("string")) -> (w371:string)
            }
            frame "10mA" {
              n177 = Multiply(x=w376, y=10.0) -> (x*y=w382:dbl)
              n178 = Divide(x=w382, y=10.0) -> (x/y=w378:dbl)
              n179 = Number To Fractional String(number=w378) -> (F-format string=w377:string)  [unwired: 3 in]
              n180 = Concatenate Strings(w377, "mA" ("string")) -> (w379:string)
            }
            frame "1mA" {
              n181 = Multiply(x=w386, y=1.0) -> (x*y=w390:dbl)
              n182 = Divide(x=w390, y=10.0) -> (x/y=w385:dbl)
              n183 = Number To Fractional String(number=w385) -> (F-format string=w384:string)  [unwired: 3 in]
              n184 = Concatenate Strings(w384, "mA" ("string")) -> (w387:string)
            }
            frame "100uA" {
              n185 = Multiply(x=w394, y=100.0) -> (x*y=w398:dbl)
              n186 = Divide(x=w398, y=10.0) -> (x/y=w393:dbl)
              n187 = Number To Fractional String(number=w393) -> (F-format string=w392:string)  [unwired: 3 in]
              n188 = Concatenate Strings(w392, "uA" ("string")) -> (w395:string)
            }
            frame "10uA" {
              n189 = Multiply(x=w402, y=10.0) -> (x*y=w406:dbl)
              n190 = Divide(x=w406, y=10.0) -> (x/y=w401:dbl)
              n191 = Number To Fractional String(number=w401) -> (F-format string=w400:string)  [unwired: 3 in]
              n192 = Concatenate Strings(w400, "uA" ("string")) -> (w403:string)
            }
            frame "1uA" {
              n193 = Multiply(x=w410, y=1.0) -> (x*y=w415:dbl)
              n194 = Divide(x=w415, y=10.0) -> (x/y=w409:dbl)
              n195 = Number To Fractional String(number=w409) -> (F-format string=w408:string)  [unwired: 3 in]
              n196 = Concatenate Strings(w408, "uA" ("string")) -> (w411:string)
            }
            frame "1A" {
              n197 = Multiply(x=w418, y=1.0) -> (x*y=w422:dbl)
              n198 = Divide(x=w422, y=10.0) -> (x/y=w417:dbl)
              n199 = Number To Fractional String(number=w417) -> (F-format string=w416:string)  [unwired: 3 in]
              n200 = Concatenate Strings(w416, "A" ("string")) -> (w419:string)
            }
          }
          n201 = property on="VI mode" class="Str"("Value"=w343) -> ()  [unwired: 2 in, 2 out]
          n202 = Pick Line(multi-line string="1A\n100mA\n10mA\n1mA\n100uA\n10uA\n1uA" ("Range"), line index=w341) -> (output string=w338:string)  [unwired: 1 in]
          n203 = property on="Range" class="Str"("Value"=w338) -> ()  [unwired: 2 in, 2 out]
          n204 = Bundle("trimmed string"=w342, "Enable"=w344, "VI mode"=w343, "output string"=w338, w335, w333, w332, w337) -> (w366:T4)  [unwired: 1 in]
        }
        "Array 2" <- w179
        "Array 3" <- w178
        "Array" <- w165
        n205 = local read "Ring"() -> (w180:u16)
        n206 = Decrement(x=w180) -> (x-1=w169:u16)
        n207 = Index Array(array=w170, index=w169) -> (element=w168:dbl)
        n208 = Index Array(array=w174, index=w169) -> (element=w173:bool)
        n209 = Index Array(array=w179, index=w169) -> (element=w171:i32)
        n210 = Index Array(array=w178, index=w169) -> (element=w172:bool)
        n211 = case shown="1" w171 {
          tunnel: ["mA" "mA" "mA" "uA" "uA" "uA" "nA"] -> w176
          frame 0, Default {
          }
          frame 1 {
          }
          frame 2 {
          }
          frame 3 {
          }
          frame 4 {
          }
          frame 5 {
          }
          frame 6 {
          }
        }
        n212 = Select(t=w176, s=w172, f="V") -> (s? t:f=w177:string)
        n213 = local write "Unit"(w177) -> ()
        n214 = case shown="True" w167 {
          selector: w167 -> [w318 _]
          tunnel: w173 -> [_ w323]
          tunnel: w172 -> [_ w322]
          tunnel: w171 -> [_ w321]
          tunnel: w168 -> [_ w320]
          tunnel: [w318 FALSE] -> w166
          frame False {
          }
          frame True {
            n215 = local write "Enable 2"(w323) -> ()
            n216 = local write "Range 2"(w321) -> ()
            n217 = local write "Output Value"(w320) -> ()
            n218 = local write "Mode"(w322) -> ()
          }
        }
      }
      frame True {
        n219 = property on="Auto\ncalibration \nmode" class="Bool (strict)"() -> ("Value"=w425:bool)  [unwired: 2 in, 2 out]
        n220 = case shown="True" w425 {
          tunnel: w429 -> [w456 w484]
          tunnel: [w454 w482] -> w428
          tunnel: [w432 w481] -> w427
          tunnel: w424 -> [w455 w483]
          frame True {
            n221 = property on="CH1\nCali mode" class="Bool (strict)"() -> ("Value"=w449:bool)  [unwired: 2 in, 2 out]
            n222 = local read "VISA resource \n2000(COM7)"() -> (w450:refnum<visa-resource-name>)
            n223 = case shown="False" w449 {
              tunnel: [w474 "1" ("string")] -> w448
              frame False {
                n224 = property on="CH2\nCali mode" class="Bool (strict)"() -> ("Value"=w473:bool)  [unwired: 2 in, 2 out]
                n225 = case shown="False" w473 {
                  tunnel: [w476 "2" ("string")] -> w474
                  frame False {
                    n226 = property on="CH3\nCali mode" class="Bool (strict)"() -> ("Value"=w475:bool)  [unwired: 2 in, 2 out]
                    n227 = case shown="False" w475 {
                      tunnel: ["4" ("string") "3" ("string")] -> w476
                      frame False {
                      }
                      frame True {
                      }
                    }
                  }
                  frame True {
                  }
                }
              }
              frame True {
              }
            }
            n228 = property on="Auto\ncalibration \nmode" class="Bool (strict)"() -> ("Value"=w453:bool)  [unwired: 2 in, 2 out]
            n229 = property on="OUTPUT_F\nmode" class="Bool (strict)"() -> ("Value"=w452:bool)  [unwired: 2 in, 2 out]
            n230 = property on="INPUT_F\nmode" class="Bool (strict)"() -> ("Value"=w451:bool)  [unwired: 2 in, 2 out]
            n231 = local read "Input calibration parameter"() -> (w446:string)
            n232 = local read "Output calibration parameter"() -> (w447:string)
            n233 = call "calibration sub_VI.vi"("VISA resource ESP32(COM4)"=w456, "Auto \ncalibration \nmode"=w453, "OUTPUT_F\nmode"=w452, "INPUT_F\nmode"=w451, "VISA resource \n2000(COM9)"=w450, "ESP32 error in"=w455, "Calibration \nChannel"=w448, "Ouput calibration\nparameter"=w447, "Input calibration\nparameter"=w446) -> ("VISA resource ESP32(COM4) 2"=w454:refnum<visa-resource-name>, "Calibration TX"=w444:string, "error out"=w431:errorcluster)  [unwired: 4 in]
            n234 = property on="CH1\nCali mode" class="Bool (strict)"() -> ("Value"=w445:bool)  [unwired: 2 in, 2 out]
            n235 = case shown="True" w445 {
              tunnel: w444 -> [w460 w472]
              tunnel: w431 -> [w457 w471]
              tunnel: [w458 w471] -> w430
              frame False {
                n236 = property on="CH2\nCali mode" class="Bool (strict)"() -> ("Value"=w459:bool)  [unwired: 2 in, 2 out]
                n237 = case shown="True" w459 {
                  tunnel: w460 -> [w464 w470]
                  tunnel: [w462 w469] -> w458
                  tunnel: w457 -> [w461 w469]
                  frame False {
                    n238 = property on="CH3\nCali mode" class="Bool (strict)"() -> ("Value"=w463:bool)  [unwired: 2 in, 2 out]
                    n239 = case shown="True" w463 {
                      tunnel: w464 -> [w466 w468]
                      tunnel: [w465 w467] -> w462
                      tunnel: w461 -> [w465 w467]
                      frame False {
                        n240 = local write "CH4 Calibration TX"(w466) -> ()
                      }
                      frame True {
                        n241 = local write "CH3 Calibration TX"(w468) -> ()
                      }
                    }
                  }
                  frame True {
                    n242 = local write "CH2 Calibration TX"(w470) -> ()
                  }
                }
              }
              frame True {
                n243 = local write "CH1 Calibration TX"(w472) -> ()
              }
            }
            n244 = property on="Write \nmode" class="Bool (strict)"(error in=w430, "Value"=FALSE ("Write mode")) -> (error out=w441:errorcluster)  [unwired: 1 in, 1 out]
            n245 = property on="calibration \nmode" class="Bool (strict)"(error in=w441, "Value"=FALSE ("calibration mode")) -> (error out=w436:errorcluster)  [unwired: 1 in, 1 out]
            n246 = property on="CH1\nCali mode" class="Bool (strict)"(error in=w436, "Value"=FALSE ("Write mode")) -> (error out=w435:errorcluster)  [unwired: 1 in, 1 out]
            n247 = property on="CH2\nCali mode" class="Bool (strict)"(error in=w435, "Value"=FALSE ("calibration \nmode 2")) -> (error out=w434:errorcluster)  [unwired: 1 in, 1 out]
            n248 = property on="CH3\nCali mode" class="Bool (strict)"(error in=w434, "Value"=FALSE ("calibration \nmode 3")) -> (error out=w433:errorcluster)  [unwired: 1 in, 1 out]
            n249 = property on="CH4\nCali mode" class="Bool (strict)"(error in=w433, "Value"=FALSE ("calibration \nmode 4")) -> (error out=w432:errorcluster)  [unwired: 1 in, 1 out]
          }
          frame False {
            n250 = property on="OUTPUT_F\nmode" class="Bool (strict)"() -> ("Value"=w485:bool)  [unwired: 2 in, 2 out]
            n251 = case shown="False" w485 {
              tunnel: w484 -> [w489 w518]
              tunnel: w483 -> [w488 w517]
              tunnel: [w487 w516] -> w482
              tunnel: [w486 w515] -> w481
              frame True {
                n252 = property on="INPUT_F\nmode" class="Bool (strict)"() -> ("Value"=w490:bool)  [unwired: 2 in, 2 out]
                n253 = case shown="False" w490 {
                  tunnel: w489 -> [w492 w508]
                  tunnel: w488 -> [w491 w507]
                  tunnel: [w494 w508] -> w487
                  tunnel: [w503 w509] -> w486
                  frame False {
                    n254 = local read "Output calibration parameter"() -> (w495:string)
                    n255 = VISA Flush I/O Buffer(VISA resource name=w492, error in (no error)=w491) -> (VISA resource name out=w496:refnum<visa-resource-name>, error out=w497:errorcluster)  [unwired: 1 in]
                    n256 = VISA Write(VISA resource name=w496, write buffer=w495, error in (no error)=w497) -> (VISA resource name out=w499:refnum<visa-resource-name>, return count=w500:u32, error out=w498:errorcluster)
                    n257 = VISA Read(VISA resource name=w499, byte count=w500, error in (no error)=w498) -> (VISA resource name out=w502:refnum<visa-resource-name>, error out=w501:errorcluster)  [unwired: 2 out]
                    n258 = VISA Flush I/O Buffer(VISA resource name=w502, error in (no error)=w501) -> (VISA resource name out=w494:refnum<visa-resource-name>, error out=w493:errorcluster)  [unwired: 1 in]
                    n259 = property on="Write \nmode" class="Bool (strict)"(error in=w493, "Value"=FALSE ("Write mode")) -> (error out=w504:errorcluster)  [unwired: 1 in, 1 out]
                    n260 = property on="OUTPUT_F\nmode" class="Bool (strict)"(error in=w504, "Value"=FALSE ("calibration mode 2")) -> (error out=w503:errorcluster)  [unwired: 1 in, 1 out]
                  }
                  frame True {
                    n261 = property on="Write \nmode" class="Bool (strict)"(error in=w507, "Value"=FALSE ("Write mode")) -> (error out=w511:errorcluster)  [unwired: 1 in, 1 out]
                    n262 = property on="OUTPUT_F\nmode" class="Bool (strict)"(error in=w511, "Value"=FALSE ("calibration mode 2")) -> (error out=w510:errorcluster)  [unwired: 1 in, 1 out]
                    n263 = property on="INPUT_F\nmode" class="Bool (strict)"(error in=w510, "Value"=FALSE ("Write mode")) -> (error out=w509:errorcluster)  [unwired: 1 in, 1 out]
                  }
                }
              }
              frame False {
                n264 = property on="INPUT_F\nmode" class="Bool (strict)"() -> ("Value"=w519:bool)  [unwired: 2 in, 2 out]
                n265 = case shown="True" w519 {
                  tunnel: w518 -> [w523 w560]
                  tunnel: w517 -> [w522 w559]
                  tunnel: [w521 w562] -> w516
                  tunnel: [w520 w564] -> w515
                  frame False {
                    n266 = property on="WRITE\nString" class="Str"() -> ("Value"=w525:string)  [unwired: 2 in, 2 out]
                    n267 = VISA Write(VISA resource name=w523, write buffer=w525, error in (no error)=w522) -> (VISA resource name out=w527:refnum<visa-resource-name>, error out=w528:errorcluster)  [unwired: 1 out]
                    n268 = while {
                      shift-right: [w548] -> w521
                      shift-left: w527 -> [w546]
                      shift-right: [w547] -> w526
                      shift-left: w528 -> [w543]
                      shift-right: [w533] -> _
                      shift-left: "" -> [w534]
                      i -> [w532]
                      stop <- w535 stop-if-true
                      n269 = property class="Instr"(reference=w546, error in=w543) -> (reference out=w545:refnum<visa-resource-name>, error out=w544:errorcluster, "Serial Settings:Number of Bytes at Serial Port"=w531:u32)
                      n270 = Wait (ms)(milliseconds to wait=u32 1) -> ()  [unwired: 1 out]
                      n271 = VISA Read(VISA resource name=w545, byte count=w531, error in (no error)=w544) -> (VISA resource name out=w548:refnum<visa-resource-name>, read buffer=w530:string, error out=w547:errorcluster)  [unwired: 1 out]
                      n272 = Match Pattern(string=w530, regular expression="\n") -> (offset past match=w540:i32)  [unwired: 1 in, 3 out]
                      n273 = Greater?(x=w532, y=5000) -> (0:w536:bool)
                      n274 = Not Equal?(x=w540, y=-1) -> (x != y?=w538:bool)
                      n275 = Concatenate Strings(w534, w530) -> (w533:string)
                      n276 = Compound Arithmetic op=OR(w538, w536) -> (w535:bool)
                    }
                    n277 = property on="Write \nmode" class="Bool (strict)"(error in=w526, "Value"=FALSE ("Write mode")) -> (error out=w520:errorcluster)  [unwired: 1 in, 1 out]
                  }
                  frame True {
                    n278 = VISA Flush I/O Buffer(VISA resource name=w560, error in (no error)=w559) -> (VISA resource name out=w551:refnum<visa-resource-name>, error out=w552:errorcluster)  [unwired: 1 in]
                    n279 = disable-structure shown="Enabled" {
                      disable-tunnel: w552 -> [_ w612]
                      disable-tunnel: w551 -> [_ w611]
                      disable-tunnel: [_ w610] -> w550
                      disable-tunnel: [_ w609] -> w549
                      frame Disabled {
                        n280 = local read "Input Calibration parameter path  - Current"() -> (w608:path)
                        n281 = local read "Input FIle \nCalibation Channel"() -> (w607:u16)
                        n282 = local read "Input Calibration parameter path  - Voltage"() -> ()  [unwired: 1 out]
                        n283 = Number To Decimal String(number=w607, width (-)=i16 1) -> (decimal integer string=w606:string)
                        n284 = call-poly <vilib>:"Read Delimited Spreadsheet.vi"("file path (dialog if empty)"=w608, "delimiter (\\t)"="," ("delimiter (\\t)")) -> ()  [unwired: 8 in, 6 out]
                        n285 = call-poly <vilib>:"Read Delimited Spreadsheet.vi"("delimiter (\\t)"="," ("delimiter (\\t)")) -> ("all rows"=w598:dbl[][])  [unwired: 9 in, 5 out]
                        n286 = Concatenate Strings("FILE" ("string"), w606, " " ("string")) -> (→"concatenated string":string)
                        n287 = Index Array(array=w598, index (col)=1 ("disabled index (col)")) -> ()  [unwired: 1 in, 1 out]
                        n288 = Index Array(array=w598, index (col)=0 ("disabled index (col)")) -> (element=w574:dbl[])  [unwired: 1 in]
                        n289 = Array Subset(array=w574, index=0, length=7) -> (w593:dbl[])
                        n290 = Array Subset(array=w574, index=14, length=7) -> (w575:dbl[])
                        n291 = Array Subset(array=w574, index=7, length=7) -> (w584:dbl[])
                        n292 = Array To Spreadsheet String(delimiter (Tab)=",", array=w593, 3:"%f" ("format string")) -> (spreadsheet string=w588:string)
                        n293 = Array To Spreadsheet String(delimiter (Tab)=",", array=w575, 3:"%f" ("format string")) -> (spreadsheet string=w569:string)
                        n294 = Array To Spreadsheet String(delimiter (Tab)=",", array=w584, 3:"%f" ("format string")) -> (spreadsheet string=w587:string)
                        n295 = call <vilib>:"Trim Whitespace.vi"("string"=w588) -> ("trimmed string"=w589:string)  [unwired: 1 in]
                        n296 = call <vilib>:"Trim Whitespace.vi"("string"=w587) -> ("trimmed string"=w586:string)  [unwired: 1 in]
                        n297 = call <vilib>:"Trim Whitespace.vi"("string"=w569) -> ("trimmed string"=w570:string)  [unwired: 1 in]
                        n298 = property on="concatenated string" class="Str"() -> ("Value"=w567:string)  [unwired: 2 in, 2 out]
                        n299 = Concatenate Strings(w567, "*" ("string"), w589, "," ("string")) -> (→"concatenated string 2":string)
                        n300 = Concatenate Strings(w586, "," ("string")) -> (→"concatenated string 3":string)  [unwired: 1 in]
                        n301 = Concatenate Strings(w570, ";" ("string")) -> (→"concatenated string 4":string)  [unwired: 1 in]
                        n302 = local read "Input calibration parameter"() -> ()  [unwired: 1 in]
                      }
                      frame Enabled {
                        n303 = stacked-sequence {
                          seq-local: [w616 _ _ _] -> [_ w677 _ _]
                          seq-local: [w615 _ _ _] -> [_ w676 _ _]
                          seq-local: [_ w675 _ _] -> [_ _ w738 _]
                          seq-local: [_ w674 _ _] -> [_ _ w737 _]
                          seq-local: [_ _ w735 _] -> [_ _ _ w797]
                          seq-local: [_ _ w734 _] -> [_ _ _ w796]
                          tunnel: w612 -> [w614 _ _ _]
                          tunnel: w611 -> [w613 _ _ _]
                          tunnel: [_ _ _ w795] -> w610
                          tunnel: [_ _ _ w794] -> w609
                          frame #0 {
                            n304 = local read "Input Calibration parameter path  - Voltage"() -> (w619:path)
                            n305 = call-poly <vilib>:"Read Delimited Spreadsheet.vi"("file path (dialog if empty)"=w619, "format (%.3f)"="%.12f", "delimiter (\\t)"="," ("delimiter (\\t)")) -> ("all rows"=w621:dbl[][])  [unwired: 7 in, 5 out]
                            n306 = Index Array(array=w621, index (col)=0 ("disabled index (col)")) -> (element=w617:dbl[])  [unwired: 1 in]
                            n307 = for {
                              N: 3 -> [_]
                              tunnel: w617 -> [w633]
                              tunnel: [w626] -> w615
                              tunnel: [w629] -> w616
                              tunnel: w614 -> [w628]
                              tunnel: w613 -> [w627]
                              i -> [w630]
                              n308 = Multiply(x=7, y=w630) -> (x*y=w631:i32)
                              n309 = case shown="3, Default" w630 {
                                tunnel: w633 -> [w640 _ w654 w666]
                                tunnel: w631 -> [w639 _ w653 w665]
                                tunnel: [w636 "" w650 w662] -> w624
                                frame 0 {
                                n310 = Array Subset(array=w640, index=w639, length=7) -> (w641:dbl[])
                                n311 = Array To Spreadsheet String(delimiter (Tab)=",", array=w641, 3:"%f" ("format string")) -> (spreadsheet string=w642:string)
                                n312 = call <vilib>:"Trim Whitespace.vi"("string"=w642) -> ("trimmed string"=w643:string)  [unwired: 1 in]
                                n313 = property on="FILE" class="Str"() -> ("Value"=w638:string)  [unwired: 2 in, 2 out]
                                n314 = Concatenate Strings(w638, "*" ("string"), w643, "," ("string"), "\n") -> (w636:string)
                                }
                                frame 3, Default {
                                }
                                frame 1 {
                                n315 = Array Subset(array=w654, index=w653, length=7) -> (w655:dbl[])
                                n316 = Array To Spreadsheet String(delimiter (Tab)=",", array=w655, 3:"%f" ("format string")) -> (spreadsheet string=w656:string)
                                n317 = call <vilib>:"Trim Whitespace.vi"("string"=w656) -> ("trimmed string"=w657:string)  [unwired: 1 in]
                                n318 = property on="FILE" class="Str"() -> ("Value"=w652:string)  [unwired: 2 in, 2 out]
                                n319 = Concatenate Strings(w652, w657, "," ("string"), "\n") -> (w650:string)
                                }
                                frame 2 {
                                n320 = Array Subset(array=w666, index=w665, length=7) -> (w667:dbl[])
                                n321 = Array To Spreadsheet String(delimiter (Tab)=",", array=w667, 3:"%f" ("format string")) -> (spreadsheet string=w668:string)
                                n322 = call <vilib>:"Trim Whitespace.vi"("string"=w668) -> ("trimmed string"=w669:string)  [unwired: 1 in]
                                n323 = property on="FILE" class="Str"() -> ("Value"=w664:string)  [unwired: 2 in, 2 out]
                                n324 = Concatenate Strings(w664, w669, ";" ("string"), "\n") -> (w662:string)
                                }
                              }
                              n325 = local write "Input calibration parameter"(w624) -> ()
                              n326 = VISA Write(VISA resource name=w627, write buffer=w624, error in (no error)=w628) -> (VISA resource name out=w629:refnum<visa-resource-name>, error out=w625:errorcluster)  [unwired: 1 out]
                              n327 = flat-sequence {
                                tunnel: [w634] -> w626
                                tunnel: w625 -> [w634]
                                frame #0 {
                                n328 = Wait (ms)(milliseconds to wait=u32 1000) -> ()  [unwired: 1 out]
                                }
                              }
                            }
                          }
                          frame #1 {
                            n329 = local read "Input Calibration parameter path  - Voltage"() -> (w680:path)
                            n330 = call-poly <vilib>:"Read Delimited Spreadsheet.vi"("file path (dialog if empty)"=w680, "format (%.3f)"="%.12f", "delimiter (\\t)"="," ("delimiter (\\t)")) -> ("all rows"=w682:dbl[][])  [unwired: 7 in, 5 out]
                            n331 = Index Array(array=w682, index (col)=1 ("disabled index (col)")) -> (element=w678:dbl[])  [unwired: 1 in]
                            n332 = for {
                              N: 3 -> [_]
                              tunnel: w678 -> [w694]
                              tunnel: w676 -> [w690]
                              tunnel: w677 -> [w689]
                              tunnel: [w686] -> w674
                              tunnel: [w688] -> w675
                              i -> [w691]
                              n333 = Multiply(x=7, y=w691) -> (x*y=w692:i32)
                              n334 = case shown="3, Default" w691 {
                                tunnel: w694 -> [w701 w713 w725 _]
                                tunnel: w692 -> [w700 w712 w724 _]
                                tunnel: [w698 w709 w721 ""] -> w685
                                frame 0 {
                                n335 = Array Subset(array=w701, index=w700, length=7) -> (w702:dbl[])
                                n336 = Array To Spreadsheet String(delimiter (Tab)=",", array=w702, 3:"%f" ("format string")) -> (spreadsheet string=w703:string)
                                n337 = call <vilib>:"Trim Whitespace.vi"("string"=w703) -> ("trimmed string"=w704:string)  [unwired: 1 in]
                                n338 = property on="FILE" class="Str"() -> ("Value"=w697:string)  [unwired: 2 in, 2 out]
                                n339 = Concatenate Strings(w697, w704, "," ("string"), "\n") -> (w698:string)
                                }
                                frame 1 {
                                n340 = Array Subset(array=w713, index=w712, length=7) -> (w714:dbl[])
                                n341 = Array To Spreadsheet String(delimiter (Tab)=",", array=w714, 3:"%f" ("format string")) -> (spreadsheet string=w715:string)
                                n342 = call <vilib>:"Trim Whitespace.vi"("string"=w715) -> ("trimmed string"=w716:string)  [unwired: 1 in]
                                n343 = property on="FILE" class="Str"() -> ("Value"=w711:string)  [unwired: 2 in, 2 out]
                                n344 = Concatenate Strings(w711, w716, "," ("string"), "\n") -> (w709:string)
                                }
                                frame 2 {
                                n345 = Array Subset(array=w725, index=w724, length=7) -> (w726:dbl[])
                                n346 = Array To Spreadsheet String(delimiter (Tab)=",", array=w726, 3:"%f" ("format string")) -> (spreadsheet string=w727:string)
                                n347 = call <vilib>:"Trim Whitespace.vi"("string"=w727) -> ("trimmed string"=w728:string)  [unwired: 1 in]
                                n348 = property on="FILE" class="Str"() -> ("Value"=w723:string)  [unwired: 2 in, 2 out]
                                n349 = Concatenate Strings(w723, w728, ";" ("string"), "\n") -> (w721:string)
                                }
                                frame 3, Default {
                                }
                              }
                              n350 = local write "Input calibration parameter"(w685) -> ()
                              n351 = VISA Write(VISA resource name=w689, write buffer=w685, error in (no error)=w690) -> (VISA resource name out=w688:refnum<visa-resource-name>, error out=w687:errorcluster)  [unwired: 1 out]
                              n352 = flat-sequence {
                                tunnel: [w695] -> w686
                                tunnel: w687 -> [w695]
                                frame #0 {
                                n353 = Wait (ms)(milliseconds to wait=u32 1000) -> ()  [unwired: 1 out]
                                }
                              }
                            }
                          }
                          frame #2 {
                            n354 = local read "Input Calibration parameter path  - Current"() -> (w736:path)
                            n355 = call-poly <vilib>:"Read Delimited Spreadsheet.vi"("file path (dialog if empty)"=w736, "format (%.3f)"="%.12f", "delimiter (\\t)"="," ("delimiter (\\t)")) -> ("all rows"=w742:dbl[][])  [unwired: 7 in, 5 out]
                            n356 = Index Array(array=w742, index (col)=0 ("disabled index (col)")) -> (element=w739:dbl[])  [unwired: 1 in]
                            n357 = for {
                              N: 3 -> [_]
                              tunnel: w739 -> [w754]
                              tunnel: w737 -> [w750]
                              tunnel: w738 -> [w749]
                              tunnel: [w746] -> w734
                              tunnel: [w748] -> w735
                              i -> [w751]
                              n358 = Multiply(x=7, y=w751) -> (x*y=w752:i32)
                              n359 = case shown="3, Default" w751 {
                                tunnel: w754 -> [w761 w773 w785 _]
                                tunnel: w752 -> [w760 w772 w784 _]
                                tunnel: [w758 w769 w781 ""] -> w745
                                frame 0 {
                                n360 = Array Subset(array=w761, index=w760, length=7) -> (w762:dbl[])
                                n361 = Array To Spreadsheet String(delimiter (Tab)=",", array=w762, 3:"%f" ("format string")) -> (spreadsheet string=w763:string)
                                n362 = call <vilib>:"Trim Whitespace.vi"("string"=w763) -> ("trimmed string"=w764:string)  [unwired: 1 in]
                                n363 = property on="FILE" class="Str"() -> ("Value"=w757:string)  [unwired: 2 in, 2 out]
                                n364 = Concatenate Strings(w757, w764, "," ("string"), "\n") -> (w758:string)
                                }
                                frame 1 {
                                n365 = Array Subset(array=w773, index=w772, length=7) -> (w774:dbl[])
                                n366 = Array To Spreadsheet String(delimiter (Tab)=",", array=w774, 3:"%f" ("format string")) -> (spreadsheet string=w775:string)
                                n367 = call <vilib>:"Trim Whitespace.vi"("string"=w775) -> ("trimmed string"=w776:string)  [unwired: 1 in]
                                n368 = property on="FILE" class="Str"() -> ("Value"=w771:string)  [unwired: 2 in, 2 out]
                                n369 = Concatenate Strings(w771, w776, "," ("string"), "\n") -> (w769:string)
                                }
                                frame 2 {
                                n370 = Array Subset(array=w785, index=w784, length=7) -> (w786:dbl[])
                                n371 = Array To Spreadsheet String(delimiter (Tab)=",", array=w786, 3:"%f" ("format string")) -> (spreadsheet string=w787:string)
                                n372 = call <vilib>:"Trim Whitespace.vi"("string"=w787) -> ("trimmed string"=w788:string)  [unwired: 1 in]
                                n373 = property on="FILE" class="Str"() -> ("Value"=w783:string)  [unwired: 2 in, 2 out]
                                n374 = Concatenate Strings(w783, w788, ";" ("string"), "\n") -> (w781:string)
                                }
                                frame 3, Default {
                                }
                              }
                              n375 = VISA Write(VISA resource name=w749, write buffer=w745, error in (no error)=w750) -> (VISA resource name out=w748:refnum<visa-resource-name>, error out=w747:errorcluster)  [unwired: 1 out]
                              n376 = local write "Input calibration parameter"(w745) -> ()
                              n377 = flat-sequence {
                                tunnel: [w755] -> w746
                                tunnel: w747 -> [w755]
                                frame #0 {
                                n378 = Wait (ms)(milliseconds to wait=u32 1000) -> ()  [unwired: 1 out]
                                }
                              }
                            }
                          }
                          frame #3 {
                            n379 = local read "Input Calibration parameter path  - Current"() -> (w798:path)
                            n380 = call-poly <vilib>:"Read Delimited Spreadsheet.vi"("file path (dialog if empty)"=w798, "format (%.3f)"="%.12f", "delimiter (\\t)"="," ("delimiter (\\t)")) -> ("all rows"=w802:dbl[][])  [unwired: 7 in, 5 out]
                            n381 = Index Array(array=w802, index (col)=1 ("disabled index (col)")) -> (element=w799:dbl[])  [unwired: 1 in]
                            n382 = for {
                              N: 3 -> [_]
                              tunnel: w799 -> [w814]
                              tunnel: w796 -> [w810]
                              tunnel: w797 -> [w809]
                              tunnel: [w807] -> w794
                              tunnel: [w808] -> w795
                              i -> [w811]
                              n383 = Multiply(x=7, y=w811) -> (x*y=w812:i32)
                              n384 = case shown="0" w811 {
                                tunnel: w814 -> [w821 w833 w845 _]
                                tunnel: w812 -> [w820 w832 w844 _]
                                tunnel: [w818 w829 w841 ""] -> w805
                                frame 0 {
                                n385 = Array Subset(array=w821, index=w820, length=7) -> (w822:dbl[])
                                n386 = Array To Spreadsheet String(delimiter (Tab)=",", array=w822, 3:"%f" ("format string")) -> (spreadsheet string=w823:string)
                                n387 = call <vilib>:"Trim Whitespace.vi"("string"=w823) -> ("trimmed string"=w824:string)  [unwired: 1 in]
                                n388 = property on="FILE" class="Str"() -> ("Value"=w817:string)  [unwired: 2 in, 2 out]
                                n389 = Concatenate Strings(w817, w824, "," ("string"), "\n") -> (w818:string)
                                }
                                frame 1 {
                                n390 = Array Subset(array=w833, index=w832, length=7) -> (w834:dbl[])
                                n391 = Array To Spreadsheet String(delimiter (Tab)=",", array=w834, 3:"%f" ("format string")) -> (spreadsheet string=w835:string)
                                n392 = call <vilib>:"Trim Whitespace.vi"("string"=w835) -> ("trimmed string"=w836:string)  [unwired: 1 in]
                                n393 = property on="FILE" class="Str"() -> ("Value"=w831:string)  [unwired: 2 in, 2 out]
                                n394 = Concatenate Strings(w831, w836, "," ("string"), "\n") -> (w829:string)
                                }
                                frame 2 {
                                n395 = Array Subset(array=w845, index=w844, length=7) -> (w846:dbl[])
                                n396 = Array To Spreadsheet String(delimiter (Tab)=",", array=w846, 3:"%f" ("format string")) -> (spreadsheet string=w847:string)
                                n397 = call <vilib>:"Trim Whitespace.vi"("string"=w847) -> ("trimmed string"=w848:string)  [unwired: 1 in]
                                n398 = property on="FILE" class="Str"() -> ("Value"=w843:string)  [unwired: 2 in, 2 out]
                                n399 = Concatenate Strings(w843, w848, "$" ("string"), "\n") -> (w841:string)
                                }
                                frame 3, Default {
                                }
                              }
                              n400 = local write "Input calibration parameter"(w805) -> ()
                              n401 = VISA Write(VISA resource name=w809, write buffer=w805, error in (no error)=w810) -> (VISA resource name out=w808:refnum<visa-resource-name>, error out=w806:errorcluster)  [unwired: 1 out]
                              n402 = flat-sequence {
                                tunnel: [w815] -> w807
                                tunnel: w806 -> [w815]
                                frame #0 {
                                n403 = Wait (ms)(milliseconds to wait=u32 1000) -> ()  [unwired: 1 out]
                                }
                              }
                            }
                          }
                        }
                      }
                    }
                    n404 = local read "Input FIle \nCalibation Channel"() -> (w558:u16)
                    n405 = Number To Decimal String(number=w558, width (-)=i16 1) -> (decimal integer string=w557:string)
                    n406 = Concatenate Strings("FILE" ("string"), w557, " " ("string")) -> (→"FILE":string)
                    n407 = VISA Flush I/O Buffer(VISA resource name=w550, error in (no error)=w549) -> (VISA resource name out=w562:refnum<visa-resource-name>, error out=w561:errorcluster)  [unwired: 1 in]
                    n408 = property on="INPUT_F\nmode" class="Bool (strict)"(error in=w561, "Value"=FALSE ("Write mode")) -> (error out=w563:errorcluster)  [unwired: 1 in, 1 out]
                    n409 = property on="Write \nmode" class="Bool (strict)"(error in=w563, "Value"=FALSE ("Write mode")) -> (error out=w564:errorcluster)  [unwired: 1 in, 1 out]
                  }
                }
              }
            }
          }
        }
      }
    }
    n410 = local read "STOP LED"() -> (w150:bool)
    n411 = case shown="True" w150 {
      selector: w150 -> [w854 w855]
      tunnel: [w854 w855] -> w149
      frame False {
      }
      frame True {
        w870 = u16 0 items=["Channel A", "Channel B"] ("Channel (Channel A)")
        w869 = u16 0 items=["Channel A", "Channel B", "Channels A & B", "User"] ("Screen (Channels A & B)")
        w871 = enum32{"Current", "Voltage"}."Voltage" ("Source Function (Current)")
        w860 = TRUE  # Reset (True)
        w857 = TRUE  # ID Query (True)
        n412 = local read "VISA resource \n2604B(COM8)"() -> (w889:refnum<visa-resource-name>)
        n413 = call <instrlib>:"Initialize.vi"("Reset (True)"=w860, "Serial Configuration"=T3 {"Baud Rate"=115200, "Parity"=0, "Data Bits"=8, "Stop Bits"=10, "Flow Control"=0}, "Error Query (False)"=FALSE, "ID Query (True)"=w857, "VISA resource name"=w889) -> ("error out"=w887:errorcluster, "VISA resource name out"=w880:refnum<visa-resource-name>)  [unwired: 1 in, 4 out]
        n414 = local read "Channel (Channel A)"() -> (w879:T2)
        n415 = call <instrlib>:"Node Format.vi"("error in"=w887) -> ("error out"=w888:errorcluster, "Formatted Node"=w886:string)  [unwired: 1 in, 8 out]
        n416 = Equal?(x=enum32{"Channel A", "Channel B"}."Channel B", y=w879) -> (x = y?=w882:bool)
        n417 = Equal?(x=enum32{"Channel A", "Channel B"}."Channel A", y=w879) -> (x = y?=w881:bool)
        n418 = call <instrlib>:"Reset SMU.vi"("SMU B (No)"=w882, "SMU A (No)"=w881, "error in (no error)"=w888, "Node In"=w886, "VISA resource name"=w880) -> ("error out"=w883:errorcluster, "Node Out"=w885:string, "VISA resource name out"=w884:refnum<visa-resource-name>)  [unwired: 4 out]
        n419 = call <instrlib>:"Source Function.vi"("Function (Current)"=w871, "error in (no error)"=w883, "Channel (Channel A)"=w879, "Node In"=w885, "VISA resource name"=w884) -> ("error out"=w876:errorcluster, "Node Out"=w877:string, "VISA resource name out"=w878:refnum<visa-resource-name>)  [unwired: 4 out]
        n420 = call <instrlib>:"Measure Autorange.vi"("Autorange (On)"=TRUE, "error in (no error)"=w876, "Channel (Channel A)"=w879, "Node In"=w877, "VISA resource name"=w878) -> ("error out"=w909:errorcluster, "Node Out"=w908:string, "VISA resource name out"=w907:refnum<visa-resource-name>)  [unwired: 3 in, 1 out]
        n421 = call <instrlib>:"Source Level.vi"("Level (0.000)"=0.0, "Function (Current)"=w871, "error in (no error)"=w909, "Channel (Channel A)"=w879, "Node In"=w908, "VISA resource name"=w907) -> ("error out"=w890:errorcluster, "Node Out"=w894:string, "VISA resource name out"=w891:refnum<visa-resource-name>)  [unwired: 3 out]
        n422 = Equal?(x=enum32{"Current", "Voltage"}."Current", y=w871) -> (x = y?=w896:bool)
        n423 = Select(t=enum32{"Current", "Voltage"}."Voltage" ("x"), s=w896, f=enum32{"Current", "Voltage"}."Current") -> (s? t:f=w897:enum32{"Current", "Voltage"})
        n424 = call <instrlib>:"Source Limit.vi"("Limit (0.000)"=1.0, "Function (Current)"=w897, "error in (no error)"=w890, "Channel (Channel A)"=w879, "Node In"=w894, "VISA resource name"=w891) -> ("error out"=w900:errorcluster, "Node Out"=w899:string, "VISA resource name out"=w898:refnum<visa-resource-name>)  [unwired: 3 out]
        n425 = call <instrlib>:"Display Screen.vi"("Screen (Channels A & B)"=w869, "error in (no error)"=w900, "Node In"=w899, "VISA resource name"=w898) -> ("error out"=w903:errorcluster, "Node Out"=w902:string, "VISA resource name out"=w901:refnum<visa-resource-name>)  [unwired: 4 in, 1 out]
        n426 = call <instrlib>:"Display Measure Function.vi"("Function (Current)"=w871, "error in (no error)"=w903, "Channel (Channel A)"=w870, "Node In"=w902, "VISA resource name"=w901) -> ("error out"=w906:errorcluster, "Node Out"=w905:string, "VISA resource name out"=w904:refnum<visa-resource-name>)  [unwired: 3 in, 1 out]
        n427 = call <instrlib>:"Source Output Enable.vi"("Output (Off)"=TRUE, "error in (no error)"=w906, "Channel (Channel A)"=w879, "Node In"=w905, "VISA resource name"=w904) -> ("error out"=w892:errorcluster, "Node Out"=w895:string, "VISA resource name out"=w893:refnum<visa-resource-name>)  [unwired: 4 out]
        n428 = call <instrlib>:"Measure.vi"("Function (Current)"=w871, "error in (no error)"=w892, "Channel (Channel A)"=w879, "Node In"=w895, "VISA resource name"=w893) -> ("error out"=w874:errorcluster, "Node Out"=w873:string, "VISA resource name out"=w875:refnum<visa-resource-name>)  [unwired: 2 in, 2 out]
        n429 = call <instrlib>:"Source Output Enable.vi"("Output (Off)"=FALSE, "error in (no error)"=w874, "Node In"=w873, "VISA resource name"=w875) -> ("error out"=w910:errorcluster, "VISA resource name out"=w911:refnum<visa-resource-name>)  [unwired: 1 in, 5 out]
        n430 = call <instrlib>:"Close.vi"("error in (no error)"=w910, "VISA resource name"=w911) -> ()  [unwired: 10 out]
      }
    }
  }
  n431 = VISA Close(VISA resource name=w27, error in (no error)=w21) -> (error out=w20:errorcluster)
  n432 = call <vilib>:"Simple Error Handler.vi"("error in (no error)"=w20) -> ()  [unwired: 4 in, 5 out]
